vi "ToggleACTestMode.vi"(8 "error in":errorcluster) -> (0 "error out":errorcluster, 3 "Return Code":i32)   [LabVIEW 2015]
doc: "This test will toggle on and then off the AC coupling setting for all channels, needed for additional mfg. validation.\n\nThis function returns a 0 if the function completed successfully. A non-zero return code will indicate error."
uses:
  ScannerDiagDLL.dll
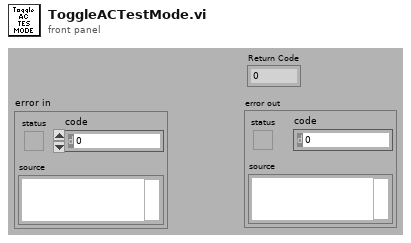
[diagram p1: front panel]
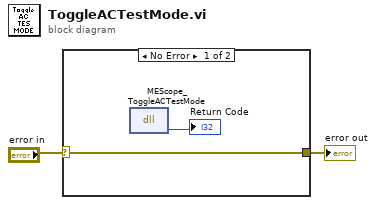
[diagram p0: block diagram]
diagram:
  n1 = case shown="No Error" "error in" {
    selector: "error in" -> [w4 w5]
    tunnel: [w4 w5] -> w1
    frame No Error {
      n2 = dll-call lib="C:/SNAPON/ModisEdge/TabletScope/Test Sequence/Code Modules/DLL/ScannerDiagDLL.dll" fn="MEScope_ToggleACTestMode"() -> ("return type"=→"Return Code":i32)  [unwired: 3 in, 2 out]
    }
    frame Error {
    }
  }
  "error out" <- w1
